vi "Power UP.vi"() -> ()   [LabVIEW 2016]
uses:
  <vilib>/LabVIEW Targets/FPGA/659XR/CustomFPGAMethods/typedefs/659XR_Clock Select Enum.ctl
  <vilib>/userdefined/Silver/nirio_resource_slv.ctl
  29x5/SubVIs/Streaming Xvcr FPGA Ref.ctl
  <vilib>/Utility/error.llb/Error Cluster From Error Code.vi
  <vilib>/rvi/errors/niLvFpgaAdjustHostInterfaceError.vi
  <vilib>/LabVIEW Targets/FPGA/659XR/CustomFPGAMethods/659XR_Read FPGA Frequency Counter.vi
  <vilib>/FPGAPlugInAG/Dynamic/niLvFpga_Close_Dynamic.vi
  <vilib>/rvi/interface/nirviReadWriteControl/nirviReadWriteControl.xnode
  <vilib>/rvi/interface/nirviMethod/nirviMethod.xnode
  <vilib>/rvi/interface/nirviCloseFPGA/nirviCloseFPGA.xnode
  6592R/SubVIs/Aurora Stream (NI 6592R) (Host).lvlib
  NiFpgaLv.dll
  <vilib>/rvi/interface/Simulation/niFpgaSimulationCallBeginRW.vi
panel:
  out "Port 2 Debug 6592R":T1
  out "Valid?":bool
  out "Frequency (Hz)":dbl format="%#_6p"
  in  "Which Clock":T2
  in  "Reset 2955":bool
  in  "Reset 6592R":bool
  in  "stop":bool
  out "Port 1 Debug 2955":T1
  out "Port 0 Debug 2955":T1
  out "Port 1 Debug 6592R":T1
  out "Port 0 Debug 6592R":T1
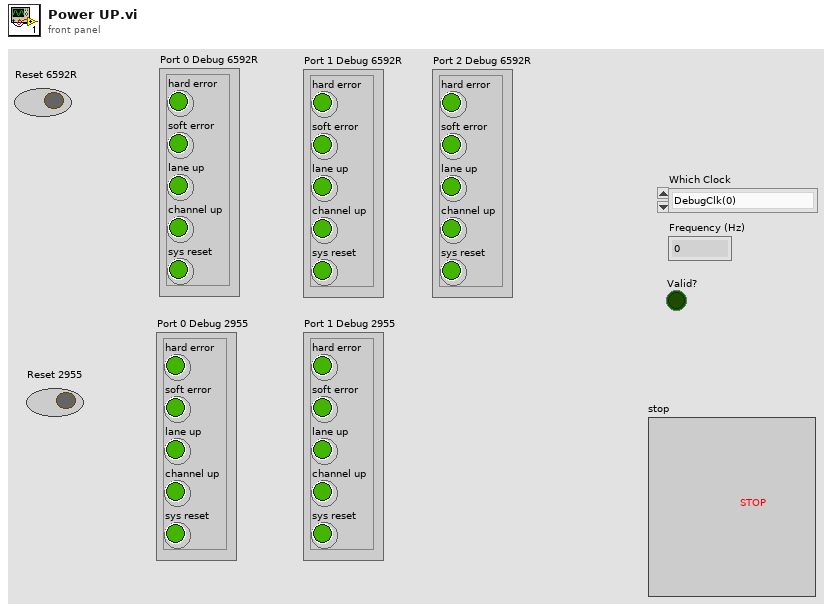
[diagram p1: front panel]
types:
  T1 = cluster{"hard error":bool, "soft error":bool, "lane up":bool, "channel up":bool, "sys reset":bool}
  T2 = typedef "659XR_Clock Select Enum.ctl" = enum16{"DebugClk(0)", "DebugClk(1)", "DebugClk(2)", "DebugClk(3)"}
  T3 = typedef "Streaming Xvcr FPGA Ref.ctl" = refnum<k20>
  T4 = typedef "nirio_resource_slv.ctl" = tag
  T5 = typedef "niUsrpRio Config v1 Host.lvlib/niUsrpRio Session.ctl" = cluster{"FPGA Interface":refnum<k20>, "RIO Interface Number":u32, "Data Clock Rate":u32, "FPGA Data Clock Rate":u32, "Global Settings Register Bus":T6, "Radio 0 Settings Register Bus":T6, "Radio 1 Settings Register Bus":T6, "Radio Settings Bus Semaphore":T7, "DB Queues":T8[], "Characterization Data Valid?":bool, "EEPROM Header":T9, "Device Data Header":T10, "EEPROM Characterization Header":T11, "Characterization Data":T12[], "FPGA Current Version":u32, "FPGA Oldest Compatible Version":u32, "Fixed Logic Current Version":u32, "Fixed Logic Oldest Compatible Version":u32, "FPGA Radio Settings Bus Current Version":u32, "FPGA Radio Settings Bus Oldest Compatible Version":u32, "FPGA Board Config Current Version":u32, "FPGA Board Config Oldest Compatible Version":u32, "Daughterboard Clock Rate":u32, "daughterboard configuration session handles":u64[]}
  T6 = typedef "niInstr Register Bus v0 Host.lvlib/Register Bus Session.ctl" = refnum<queue>
  T7 = typedef "Semaphore RefNum" = refnum<k1>
  T8 = typedef "niUsrpRio Config v1 Host.lvlib/DB Queue Reference.ctl" = refnum<queue>
  T9 = typedef "niUsrpRio Config v1 Host.lvlib/EEPROM Header.ctl" = cluster{"Checksum":u32, "Product Code":u16, "Hardware Current Version":u16, "Hardware Oldest Compatible Version":u16, "EEPROM Map Current Version":u16, "EEPROM Map Oldest Compatible Version":u16, "User Password":string, "Pointer to Factory Header":u32, "Pointer to User Header":u32, "Recommended Interval":u16, "Number of Reserved Bytes":i32, "Number of Daughterboards":u8, "Daughterboard IDs":u16[], "Daughterboard Serial Numbers":string[]}
  T10 = typedef "niUsrpRio Config v1 Host.lvlib/EEPROM Device Data Header.ctl" = cluster{"Checksum":u32, "Number of Channels":u8, "Number of Gain Settings":u16[], "Pointer to Characterization Data":u32[], "Number of Reserved Bytes":i32, "Number of Frequencies":u16[]}
  T11 = typedef "niUsrpRio Config v1 Host.lvlib/EEPROM Characterization Header.ctl" = cluster{"Checksum":u32, "Date":timestamp, "Temperature":sgl, "Misc. Info":string, "Pointer to Device Data Header":u32, "Number of Reserved Bytes":i32}
  T12 = typedef "niUsrpRio Config v1 Host.lvlib/Characterization Data.ctl" = cluster{"Gains[dB]":dbl[], "Frequencies [Hz]":dbl[], "IQ Imbalance Table":T13[], "Measured Gains[dB]":dbl[][]}
  T13 = typedef "niUsrpRio Config v1 Host.lvlib/IQ Imbalance.ctl" = cluster{"Gain Imbalance [linear]":dbl, "Phase Imbalance [radians]":dbl, "Offset":cdb}
  T14 = cluster{"Hard Error":bool, "Soft Error":bool, "Lane Up":bool, "Channel Up":bool, "Sys Reset":bool}
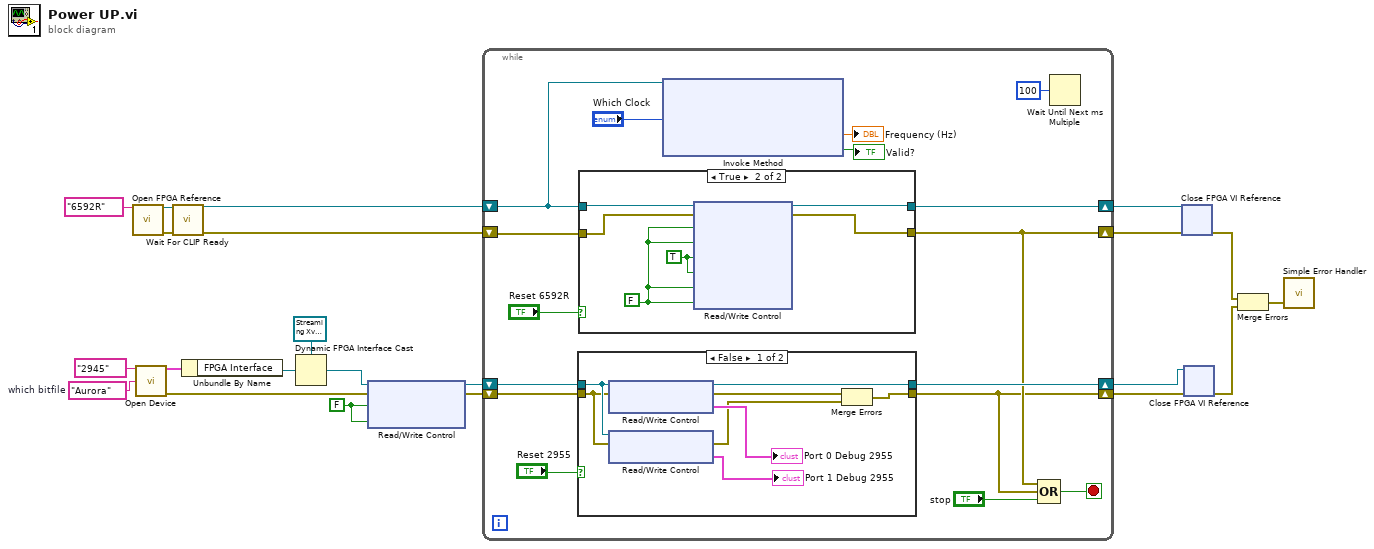
[diagram p0: block diagram]
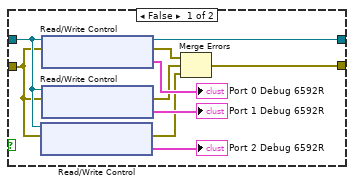
[diagram p2: hidden frame]
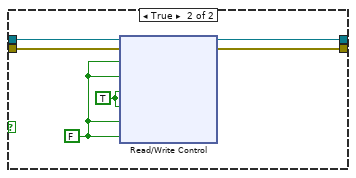
[diagram p3: hidden frame]
diagram:
  w10 = FALSE
  w14 = "Aurora"  # which bitfile
  n1 = call "Open FPGA Reference.vi"("FPGA Resource"=T4 "6592R") -> ("FPGA VI Reference Out"=w22:refnum<k20>, "error out"=w21:errorcluster)  [unwired: 13 in]
  n2 = call "Open Device.vi"("USRP RIO device"=T4 "2945", "which bitfile"=w14) -> ("niUsrpRio Session (out)"=w11:T5, "error out"=w7:errorcluster)  [unwired: 12 in]
  n3 = call "Wait For CLIP Ready.vi"("Refnum in"=w22, "error in"=w21) -> ("Refnum out"=w19:refnum<k20>, "error out"=w18:errorcluster)  [unwired: 11 in, 1 out]
  n4 = Unbundle By Name(w11) -> ("FPGA Interface"=w12:refnum<k20>)
  n5 = Dynamic FPGA Interface Cast(Session In=T3 refnum ("FPGA VI Reference Out"), Type=w12) -> (Session Out=w9:T3)
  n6 = xnode "Read/Write Control"("FPGA VI Reference In"=w9, "error in"=w7, "sfp 0.core reset"=w10, "sfp 1.core reset"=w10) -> ("FPGA VI Reference Out"=w8:T3, "error out"=w6:errorcluster)
  n7 = while {
    shift-right: [w37] -> w17
    shift-left: w19 -> [w27]
    shift-right: [w32] -> w16
    shift-left: w18 -> [w38]
    shift-right: [w30] -> w5
    shift-left: w6 -> [w36]
    shift-right: [w35] -> w4
    shift-left: w8 -> [w23]
    stop <- w33 stop-if-true
    n8 = case shown="False" "Reset 2955" {
      tunnel: w23 -> [w62 w68]
      tunnel: w36 -> [w61 w67]
      tunnel: [w58 w66] -> w35
      tunnel: [w55 w65] -> w30
      frame False {
        n9 = xnode "Read/Write Control"("FPGA VI Reference In"=w62, "error in"=w61) -> ("FPGA VI Reference Out"=w58:T3, "error out"=w57:errorcluster, "sfp 0.debug info"=→"Port 0 Debug 2955":T1)
        n10 = xnode "Read/Write Control"("FPGA VI Reference In"=w62, "error in"=w61) -> ("error out"=w56:errorcluster, "sfp 1.debug info"=→"Port 1 Debug 2955":T1)  [unwired: 1 out]
        n11 = Merge Errors(w57, w56) -> (w55:errorcluster)
      }
      frame True {
        w63 = TRUE ("sfp 0.core reset")
        w64 = FALSE
        n12 = xnode "Read/Write Control"("FPGA VI Reference In"=w68, "error in"=w67, "sfp 0.core reset"=w64, "sfp 1.core reset"=w64, "sfp 0.core reset"=w63, "sfp 1.core reset"=w63, "sfp 0.core reset"=w64, "sfp 1.core reset"=w64) -> ("FPGA VI Reference Out"=w66:T3, "error out"=w65:errorcluster)
      }
    }
    n13 = case shown="True" "Reset 6592R" {
      tunnel: w27 -> [w42 w54]
      tunnel: w38 -> [w41 w53]
      tunnel: [w46 w50] -> w37
      tunnel: [w43 w49] -> w32
      frame False {
        n14 = xnode "Read/Write Control"("FPGA VI Reference In"=w42, "error in"=w41) -> ("error out"=w39:errorcluster, "Port 2 Debug Info"=→"Port 2 Debug 6592R":T14)  [unwired: 1 out]
        n15 = xnode "Read/Write Control"("FPGA VI Reference In"=w42, "error in"=w41) -> ("FPGA VI Reference Out"=w46:refnum<k20>, "error out"=w45:errorcluster, "Port 0 Debug Info"=→"Port 0 Debug 6592R":T14)
        n16 = xnode "Read/Write Control"("FPGA VI Reference In"=w42, "error in"=w41) -> ("error out"=w44:errorcluster, "Port 1 Debug Info"=→"Port 1 Debug 6592R":T14)  [unwired: 1 out]
        n17 = Merge Errors(w45, w44, w39) -> (w43:errorcluster)
      }
      frame True {
        w52 = TRUE
        w51 = FALSE
        n18 = xnode "Read/Write Control"("FPGA VI Reference In"=w54, "error in"=w53, "Port 0 PMA Init"=w51, "Port 1 PMA Init"=w51, "Port 0 PMA Init"=w52, "Port 1 PMA Init"=w52, "Port 0 PMA Init"=w51, "Port 1 PMA Init"=w51) -> ("FPGA VI Reference Out"=w50:refnum<k20>, "error out"=w49:errorcluster)
      }
    }
    n19 = xnode "Invoke Method"("FPGA VI Reference In"=w27, "Which Clock"="Which Clock") -> ("Frequency (Hz)"=→"Frequency (Hz)":dbl, "Valid?"=→"Valid?":bool)  [unwired: 1 in, 2 out]
    n20 = Compound Arithmetic op=OR(w32, w30, "stop") -> (w33:bool)
    n21 = Wait Until Next ms Multiple(millisecond multiple=u32 100) -> ()  [unwired: 1 out]
  }
  n22 = xnode "Close FPGA VI Reference"("FPGA VI Reference In"=w17, "error in"=w16) -> ("error out"=w3:errorcluster)
  n23 = xnode "Close FPGA VI Reference"("FPGA VI Reference In"=w4, "error in"=w5) -> ("error out"=w2:errorcluster)
  n24 = Merge Errors(w3, w2) -> (w1:errorcluster)
  n25 = call <vilib>:"Simple Error Handler.vi"("error in (no error)"=w1) -> ()  [unwired: 4 in, 5 out]
